vi "Emballage_BDD_Suppression_SQL.vi"(6 "NO_DU_CARTON":string, 8 "error in (no error)":errorcluster, 9 "SN_PRODUIT":string, 10 "NO_CDEVAL":string, 11 "Table":string) -> (0 "error out":errorcluster)   [LabVIEW 2020]
uses:
  Modules/FS/60_FS_Controles/60_FS_SetGet.ctl
  <vilib>/addons/database/Connection.llb/DB Tools Open Connec (Path).vi
  <vilib>/addons/database/Connection.llb/Conn Execute.vi
  <vilib>/addons/database/Recordset.llb/Rec Destroy - Connection.vi
  <vilib>/addons/database/NI_Database_API.lvlib
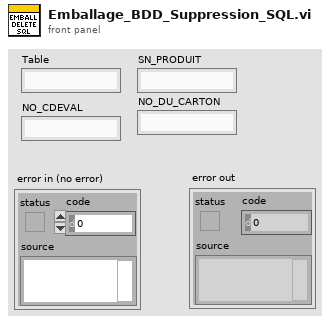
[diagram p1: front panel]
types:
  T1 = typedef "60_FS_SetGet.ctl" = enum16{"set", "get"}
  T2 = typedef "60_FS_CLT_Chemins.ctl" = cluster{"Racine_local":path, "Racine_reseau":path, "Racine_Support_Application":path, "Fichier_Journalisation":path, "Connexion_BDD_VSX":path, "Connexion_BDD_PLZ":path}
  T3 = typedef "NI_Database_API.lvlib/Conn ObjectReference.ctl" = refnum<k1>
  T4 = typedef "NI_Database_API.lvlib/Rec ObjectReference.ctl" = refnum<k1>
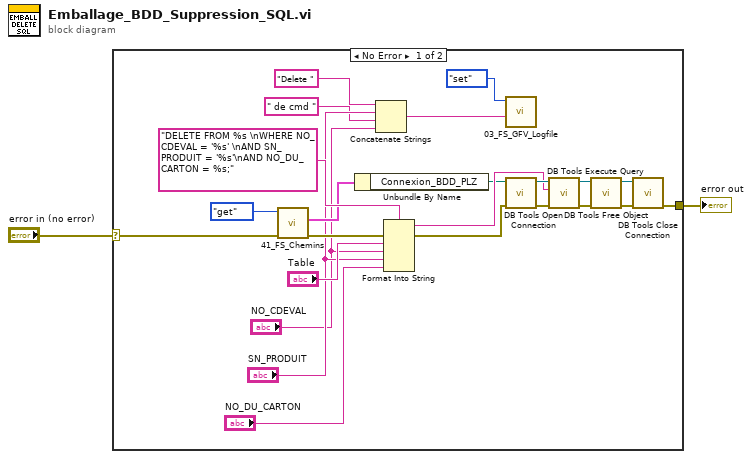
[diagram p0: block diagram]
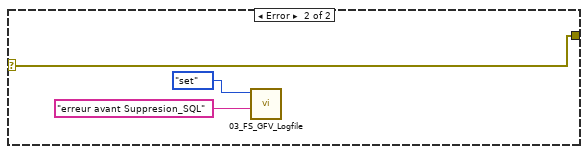
[diagram p2: hidden frame]
diagram:
  n1 = case shown="No Error" "error in (no error)" {
    selector: "error in (no error)" -> [w11 w28]
    tunnel: [w10 w28] -> w1
    frame No Error {
      n2 = call "41_FS_Chemins.vi"("error in (no error)"=w11, "SetGet"=60_FS_SetGet."get") -> ("error out"=w12:errorcluster, "CLT_Chemins_out"=w16:T2)  [unwired: 8 in]
      n3 = Unbundle By Name(w16) -> ("Connexion_BDD_PLZ"=w14:path)
      n4 = Concatenate Strings("Delete " ("chaîne"), "SN_PRODUIT", " de cmd " ("chaîne"), "NO_CDEVAL") -> (w7:string)
      n5 = Format Into String(format string="DELETE FROM %s \nWHERE NO_CDEVAL = '%s' \nAND SN_PRODUIT = '%s'\nAND NO_DU_CARTON = %s;" ("chaîne de format"), error in=w12, "Table", "NO_CDEVAL", "SN_PRODUIT", "NO_DU_CARTON") -> (resulting string=w19:string, error out=w17:errorcluster)  [unwired: 1 in]
      n6 = call "03_FS_GFV_Logfile.vi"("Chaîne"=w7, "States"=60_FS_SetGet."set") -> ()  [unwired: 8 in, 2 out]
      n7 = call-poly <vilib>:"DB Tools Open Connection.vi"("error in (no error)"=w17, "connection information"=w14) -> ("error out"=w25:errorcluster, "connection reference"=w20:T3)  [unwired: 6 in]
      n8 = call-poly <vilib>:"DB Tools Execute Query.vi"("error in (no error)"=w25, "SQL query"=w19, "connection reference"=w20) -> ("error out"=w24:errorcluster, "recordset reference"=w23:T4)  [unwired: 5 in]
      n9 = call-poly <vilib>:"DB Tools Free Object.vi"("error in (no error)"=w24, "recordset reference"=w23) -> ("error out"=w22:errorcluster, "connection reference"=w21:T3)  [unwired: 8 in]
      n10 = call <vilib>:"DB Tools Close Connection.vi"("error in (no error)"=w22, "connection reference"=w21) -> ("error out"=w10:errorcluster)  [unwired: 5 in]
    }
    frame Error {
      n11 = call "03_FS_GFV_Logfile.vi"("Chaîne"="erreur avant Suppresion_SQL", "States"=60_FS_SetGet."set") -> ()  [unwired: 8 in, 2 out]
    }
  }
  "error out" <- w1
